vi "GetClassDependencies.vi"(0 "LibReader in":refnum<class "LibReader.lvclass">, 1 "DependencyVIs":T4[](array[typedef]), 2 "Attributes":T1[](array[typedef])=[{"name"="MyU8", "type"=enum."UINT8", "dimension"=0, "typeName"="", "typePath"=path "", "visibility"=enum."Protected"}, {"name"="MyStrArray", "type"=enum."STRING", "dimension"=1, "typeName"="", "typePath"=path "", "visibility"=enum."Protected"}], 5 "error in (no error)":errorcluster) -> (14 "LibReader out":refnum<class "LibReader.lvclass">, 15 "DependencyClassPaths":path[](array[path]), 16 "IsDependencyClassPathsAByValueClass":bool[](array[boolean]), 17 "CreateClassVIsCalled":path[](array[path]), 19 "error out":errorcluster)   [LabVIEW 2014, in "LibReader.lvclass"]
uses:
  <resource>/Framework/Providers/Open_GDS/ClassProviders/LibProvider_BaseClassInterface/LibReader_class/LibReader.lvclass
  <resource>/Framework/Providers/Open_GDS/ClassProviders/Provider_BaseClassInterface/ClassReader_class/MethodDependencyType.ctl
  <resource>/Framework/Providers/Open_GDS/ClassProviders/Common/ScriptingFunctions/SubVIs/Scripting_ViDependencyType.ctl
  <resource>/Framework/Providers/Open_GDS/UML/ReversedEngineering/ReversedEngineering AttributeInfoType.ctl
  <resource>/Framework/Providers/Open_GDS/ClassProviders/Common/CommonVIs/CommonVIs_AttributeDataType.ctl
  <resource>/Framework/Providers/Open_GDS/UML/UMLEditor/UMLEditor_VisibilityType.ctl
  <resource>/Framework/Providers/Open_GDS/ClassProviders/LibProvider_BaseClassInterface/LibReader_class/LibReader.lvclass/LibReader.ctl
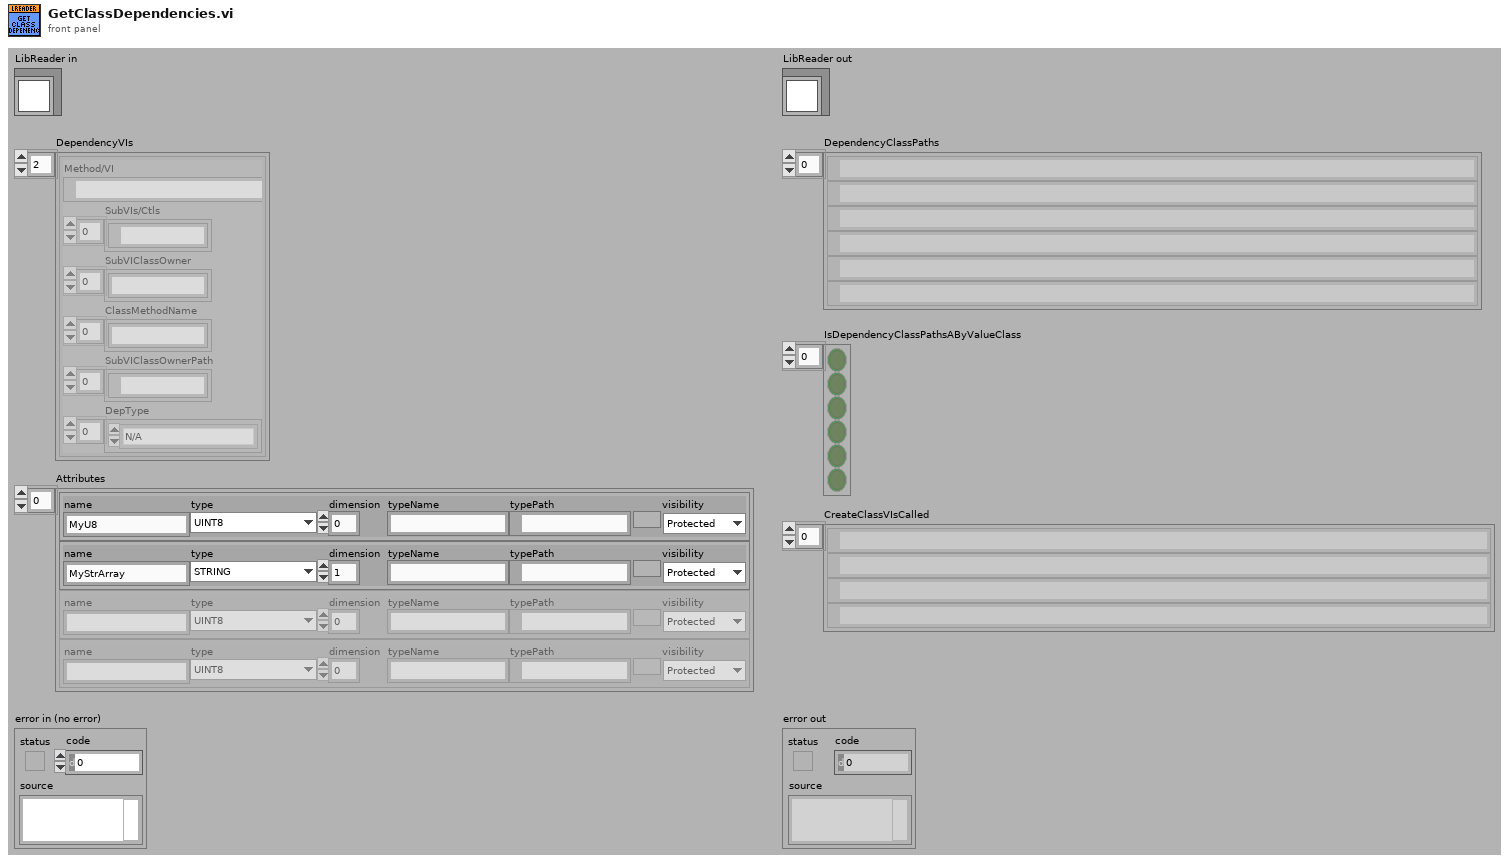
[diagram p1: front panel]
types:
  T1 = typedef "ReversedEngineering AttributeInfoType.ctl" = cluster{"name":string, "type":T2, "dimension":i32, "typeName":string, "typePath":path, "visibility":T3}
  T2 = typedef "CommonVIs_AttributeDataType.ctl" = enum16{"UINT8", "INT8", "UINT16", "INT16", "UINT32", "INT32", "UINT64", "INT64", "SGL", "DBL", "EXT", "CSG", "CDB", "CXT", "TimeStamp", "STRING", "PATH", "BOOL", "ENUM", "RefNum", "VIRefNum", "LabVIEW Class", "Cluster", "Variant", "TypeDef", "Waveform", "LabVIEW Object", "Other", "void"}
  T3 = typedef "UMLEditor_VisibilityType.ctl" = enum16{"Public", "Private", "Protected"}
  T4 = typedef "MethodDependencyType.ctl" = cluster{"Method/VI":path, "SubVIs/Ctls":path[], "SubVIClassOwner":string[], "ClassMethodName":string[], "SubVIClassOwnerPath":path[], "DepType":T5[]}
  T5 = typedef "Scripting_ViDependencyType.ctl" = enum16{"N/A", "Launches"}
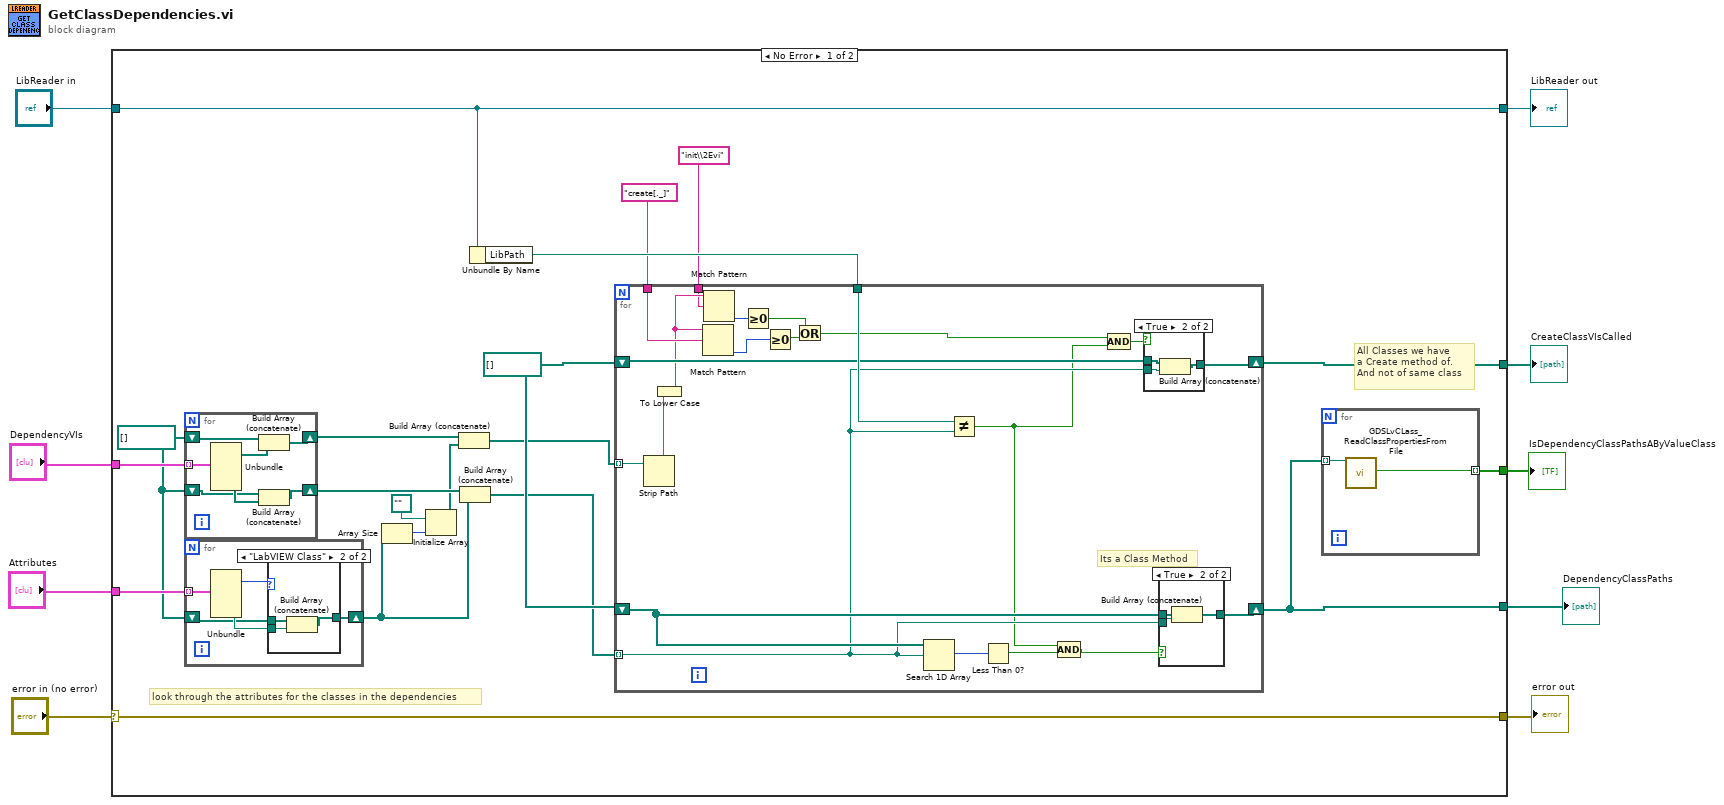
[diagram p0: block diagram]
diagram:
  n1 = case shown="No Error" "error in (no error)" {
    selector: "error in (no error)" -> [w26 w78]
    tunnel: [w26 w78] -> w8
    tunnel: [w27 w77] -> w6
    tunnel: "LibReader in" -> [w27 w77]
    tunnel: "DependencyVIs" -> [w23 _]
    tunnel: [w10 _] -> w4
    tunnel: [w12 _] -> w3
    tunnel: "Attributes" -> [w22 _]
    tunnel: [w11 _] -> w1
    frame No Error {
      w13 = path[] []
      w28 = path[] []
      # "look through the attributes for the classes in the dependencies"
      # "All Classes we have\na Create method of.\nAnd not of same class"
      n2 = for {
        tunnel: w23 -> [w76] mode=indexing
        shift-right: [w74] -> w21
        shift-left: w13 -> [w75]
        shift-right: [w71] -> w19
        shift-left: w13 -> [w70]
        n3 = Unbundle(w76) -> ("SubVIs/Ctls"=w73:path[], "SubVIClassOwnerPath"=w72:path[])  [unwired: 4 out]
        n4 = Build Array (concatenate)(w75, w73) -> (w74:path[])
        n5 = Build Array (concatenate)(w70, w72) -> (w71:path[])
      }
      n6 = for {
        tunnel: w22 -> [w65] mode=indexing
        shift-right: [w63] -> w17
        shift-left: w13 -> [w61]
        n7 = Unbundle(w65) -> ("type"=w62:T2, "typePath"=w64:path)  [unwired: 4 out]
        n8 = case shown="\"LabVIEW Class\"" w62 {
          tunnel: w61 -> [w66 w69]
          tunnel: w64 -> [_ w68]
          tunnel: [w66 w67] -> w63
          frame "UINT8", Default {
          }
          frame "LabVIEW Class" {
            n9 = Build Array (concatenate)(w69, w68) -> (w67:path[])
          }
        }
      }
      n10 = Array Size(array=w17) -> (size(s)=w16:i32)
      n11 = Initialize Array(path "" ("Path"), w16) -> (w14:path[])
      n12 = Build Array (concatenate)(w21, w14) -> (w20:path[])
      n13 = Build Array (concatenate)(w19, w17) -> (w18:path[])
      n14 = Unbundle By Name(w27) -> ("LibPath"=w29:path)
      n15 = for {
        shift-right: [w50] -> w10
        shift-left: w28 -> [w51]
        tunnel: w29 -> [w49]
        shift-right: [w46] -> w12
        shift-left: w28 -> [w47]
        tunnel: w20 -> [w43] mode=indexing
        tunnel: "create[._]" ("string") -> [w41]
        tunnel: "init\\2Evi" ("string") -> [w36]
        tunnel: w18 -> [w35] mode=indexing
        # "Its a Class Method"
        n16 = Strip Path(path=w43) -> (name=w42:string)  [unwired: 1 out]
        n17 = To Lower Case(string=w42) -> (all lower case string=w40:string)
        n18 = Match Pattern(string=w40, regular expression=w41) -> (offset past match=w45:i32)  [unwired: 1 in, 3 out]
        n19 = Match Pattern(string=w40, regular expression=w36) -> (offset past match=w39:i32)  [unwired: 1 in, 3 out]
        n20 = Greater Or Equal To 0?(x=w39) -> (x >= 0?=w37:bool)
        n21 = Greater Or Equal To 0?(x=w45) -> (x >= 0?=w44:bool)
        n22 = Or(x=w37, y=w44) -> (x .or. y?=w38:bool)
        n23 = Search 1D Array(1D array=w51, element=w35) -> (index of element=w52:i32)  [unwired: 1 in]
        n24 = Not Equal?(x=w49, y=w35) -> (x != y?=w32:bool)
        n25 = Less Than 0?(x=w52) -> (x < 0?=w34:bool)
        n26 = Compound Arithmetic op=AND(w32, w34) -> (w33:bool)
        n27 = Compound Arithmetic op=AND(w38, w32) -> (w48:bool)
        n28 = case shown="True" w48 {
          tunnel: w47 -> [w53 w56]
          tunnel: w35 -> [_ w55]
          tunnel: [w53 w54] -> w46
          frame False {
          }
          frame True {
            n29 = Build Array (concatenate)(w56, w55) -> (w54:path[])
          }
        }
        n30 = case shown="True" w33 {
          tunnel: w51 -> [w57 w60]
          tunnel: [w57 w59] -> w50
          tunnel: w35 -> [_ w58]
          frame False {
          }
          frame True {
            n31 = Build Array (concatenate)(w60, w58) -> (w59:path[])
          }
        }
      }
      n32 = for {
        tunnel: w10 -> [w31] mode=indexing
        tunnel: [w30] -> w11 mode=indexing
        n33 = call <resource>:"GDSLvCLass_ReadClassPropertiesFromFile.vi"("LvClassPathIn"=w31) -> ("DataFlowClass"=w30:bool)  [unwired: 15 in, 3 out]
      }
    }
    frame Error {
    }
  }
  "error out" <- w8
  "LibReader out" <- w6
  "DependencyClassPaths" <- w4
  "CreateClassVIsCalled" <- w3
  "IsDependencyClassPathsAByValueClass" <- w1
